vi "LINX - Interactions DHT11.vi"() -> ()   [LabVIEW 2020]
doc: "DHT11 Temperature and Humidity Sensor\n\nThis example demonstrates how to read the DHT11 sensor included in the LabVIEW Interactions Parts Kit. Make sure\nthat you are using the correct firmware version so the DHT functions are supported. \n\nInstructions:\n1. Select the COM Port associated with the LINX device\n2. Enter the DHT Data Pin\n3. Click the Run Arrow."
uses:
  vi.lib/MakerHub/LINX/Public/Utilities/Open Serial.vi
  vi.lib/MakerHub/LINX/LMH-LINX.lvlib
  vi.lib/MakerHub/LINX/Private/Device/Device.lvlib
  vi.lib/MakerHub/LINX/Public/Sensors/Digilent/Interaction Parts Kit/Interaction Parts Kit.lvlib
panel:
  out "DHT Readings":T1
  in  "DHT Data Pin":u8=26
  out "Loop Rate (Hz)":u32
  in  "Serial Port":refnum<visa-resource-name>="N/A"
  in  "Stop Button":bool
  # "DHT11 Temperature and Humidity Sensor\n\nThis example demonstrates how to read the DHT11 sensor included in the LabVIEW Interactions Parts Kit.  \nMake sure that you are using the correct firmware version so the DHT functions are supported. \n\nInstructions:\n1. Select the COM Port associated with the LINX device\n2. Enter the DHT Data Pin\n3. Click the Run Arrow."
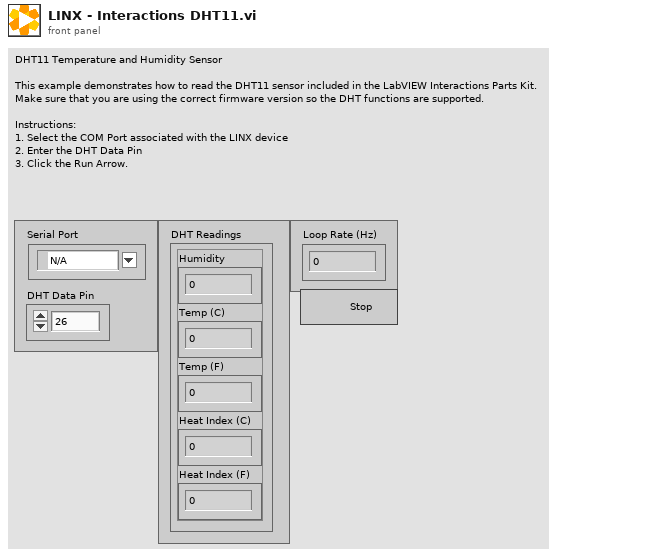
[diagram p1: front panel]
types:
  T1 = cluster{"Humidity":u8, "Temp (C)":u8, "Temp (F)":u8, "Heat Index (C)":u8, "Heat Index (F)":u8}
  T2 = typedef "LMH-LINX.lvlib/LINX Ref.ctl" = cluster{"IO":T3, "Interface":T4, "LINX Device Config":T5}
  T3 = typedef "LMH-LINX.lvlib/Platform.ctl" = enum16{"Remote", "Local"}
  T4 = typedef "LMH-LINX.lvlib/Interface.ctl" = enum16{"Serial", "TCP"}
  T5 = typedef "Device.lvlib/LINX Device Config.ctl" = cluster{"Interface":T4, "COM Port":refnum<visa-resource-name>, "TCP Configuration":T6, "Device Family":u8, "Device ID":u8, "Device Name":string, "TCP Ref":refnum<k5>, "Channels":T7}
  T6 = typedef "Device.lvlib/TCP Config.ctl" = cluster{"IP Address":string, "Port":u16}
  T7 = typedef "LMH-LINX.lvlib/Channels.ctl" = cluster{"DI":u8[], "DO":u8[], "AI":u8[], "AO":u8[], "PWM":u8[], "QE":u8[], "UART":u8[], "I2C 2":u8[], "SPI":u8[], "CAN":u8[], "Servo":u8[], "AI Ref (V)":dbl, "AI Resolution (Bits)":u8, "AO Ref (V)":dbl, "AO Resolution (Bits)":u8}
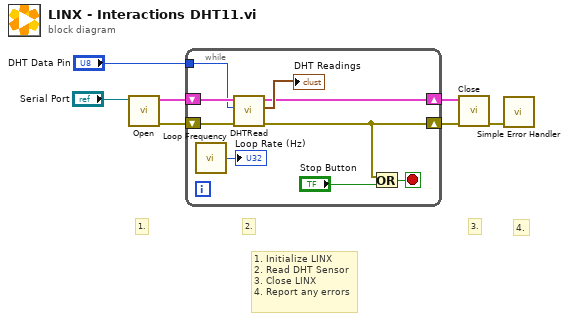
[diagram p0: block diagram]
diagram:
  # "4."
  # "1."
  # "2."
  # "3."
  # "1. Initialize LINX\n2. Read DHT Sensor\n3. Close LINX\n4. Report any errors"
  n1 = call-poly "Open.vi"("Serial Port"="Serial Port") -> ("Error Out"=w6:errorcluster, "LINX Resource"=w7:T2)  [unwired: 8 in, 1 out]
  n2 = while {
    shift-right: [w13] -> w5
    shift-left: w7 -> [w16]
    shift-right: [w9] -> w4
    shift-left: w6 -> [w15]
    tunnel: "DHT Data Pin" -> [w8]
    stop <- w11 stop-if-true
    n3 = call "Loop Frequency.vi"() -> ("Loop Rate (Hz)"=→"Loop Rate (Hz)":u32)
    n4 = call "DHTRead.vi"("Error In"=w15, "DHT Data Pin"=w8, "LINX Resource"=w16) -> ("Error Out"=w9:errorcluster, "DHT Readings"=→"DHT Readings":T1, "LINX Resource"=w13:T2)  [unwired: 6 in]
    n5 = Or(x=w9, y="Stop Button") -> (x .or. y?=w11:bool)
  }
  n6 = call "Close.vi"("Error In"=w4, "LINX Resource"=w5) -> ("Error Out"=w1:errorcluster)  [unwired: 9 in]
  n7 = call <vilib>:"Simple Error Handler.vi"("error in (no error)"=w1) -> ()  [unwired: 4 in, 5 out]
